vi "Thermal Chamber Controller_DQMH_Action Update Heater State-test_harness-Caraya.vi"(8 "error in (no error)":errorcluster) -> (0 "error out":errorcluster)   [LabVIEW 2018]
doc: "The harness VI is executed for every test case. InstaCoverage passes the test case ID before the execution of the test case in the <b>test case ID</b> input and reads the <b>result</b> output after the execution. If the result is TRUE and no error happens during the execution, then the test case is evaluated as PASSED. If the result is false and no error happens during the execution, then the test case is evaluated as FAILED. Otherwise the test case is evaluated as ERROR.\n\nThe result of the test suite will be PASSED (FAILED) if all (at least one) test cases are PASSED (FAILED). If at least one test case in the test suite has the ERROR result, then the test suite will have ERROR result.\n\n<b>Note: </b>Don't change the connector pane of this VI.\n\nSee the Help Document for more information. (<b>Help</b> > <b>IncQuery Labs</b> > <b>InstaCoverage</b> > <b>InstaCoverage Help...</b>)"
uses:
  <vilib>/addons/_JKI Toolkits/Caraya/classes/Assert/Assert True.vi
  Libraries/Thermal Chamber Controller_DQMH/Thermal Chamber Controller_DQMH.lvlib
  <vilib>/addons/_JKI Toolkits/Caraya/classes/Test/Test.lvclass
  <vilib>/addons/_JKI Toolkits/Caraya/classes/Assert/Assert.lvclass
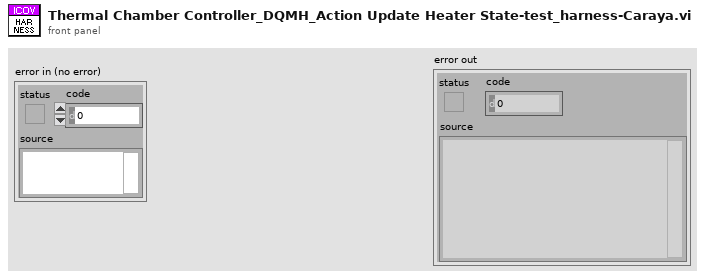
[diagram p1: front panel]
types:
  T1 = typedef "Thermal Chamber Controller_DQMH.lvlib/Heater State--enum.ctl" = enum16{"Heater Enabled", "Heater Disabled"}
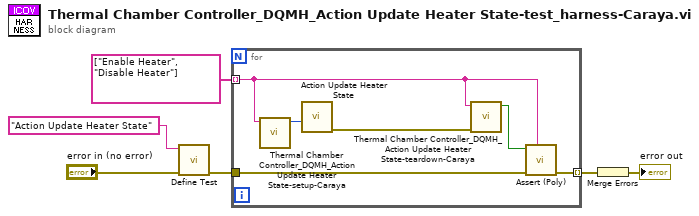
[diagram p0: block diagram]
diagram:
  n1 = call <vilib>:"Define Test.vi"("error in (no error)"="error in (no error)", "Label (VI Title)"="Action Update Heater State") -> ("error out"=w3:errorcluster)  [unwired: 9 in]
  n2 = for {
    tunnel: string[] ["Enable Heater", "Disable Heater"] -> [w8] mode=indexing
    tunnel: w3 -> [w9]
    tunnel: [w7] -> w1 mode=indexing
    n3 = call "Thermal Chamber Controller_DQMH_Action Update Heater State-setup-Caraya.vi"("test case ID"=w8) -> ("Heater State"=w11:T1)  [unwired: 10 in]
    n4 = call "Action Update Heater State.vi"("Heater State"=w11) -> ("error out"=w12:errorcluster)  [unwired: 10 in]
    n5 = call "Thermal Chamber Controller_DQMH_Action Update Heater State-teardown-Caraya.vi"("error in (no error)"=w12, "test case ID"=w8) -> ("result"=w10:bool)  [unwired: 9 in]
    n6 = call-poly <vilib>:"Assert (Poly).vi"("Label"=w8, "error in (no error)"=w9, "True?"=w10) -> ("error out"=w7:errorcluster)  [unwired: 8 in]
  }
  n7 = Merge Errors(w1) -> (→"error out":errorcluster)
